vi "SetCommand.vi"(0 "reference in":refnum<class "Panel.lvclass">, 1 "Command.lvclass":refnum<class "Command.lvclass">, 5 "error in (no error)":errorcluster) -> (14 "reference out":refnum<class "Panel.lvclass">, 19 "error out":errorcluster)   [LabVIEW 2013]
uses:
  Panel.lvclass
  Command_class/Command.lvclass
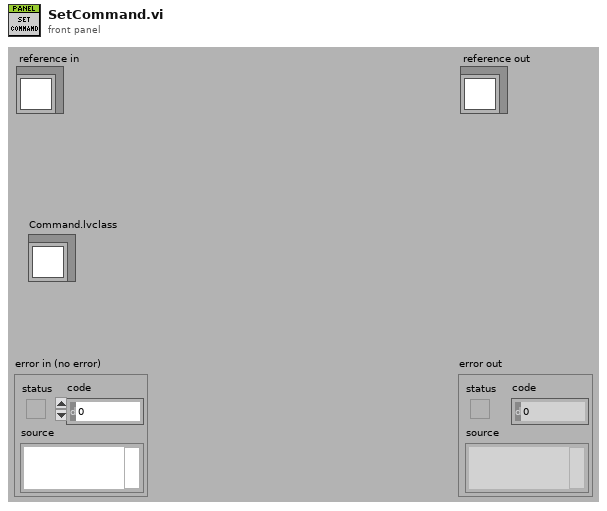
[diagram p1: front panel]
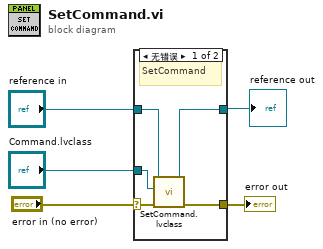
[diagram p0: block diagram]
diagram:
  n1 = case shown="无错误" "error in (no error)" {
    selector: "error in (no error)" -> [w7 w12]
    tunnel: [w6 w12] -> w4
    tunnel: [w9 w11] -> w2
    tunnel: "reference in" -> [w10 w11]
    tunnel: "Command.lvclass" -> [w8 _]
    frame No Error {
      # "SetCommand"
      n2 = call-dynamic "SetCommand.lvclass.vi"("error in (no error)"=w7, "Command.lvclass"=w8, "reference in"=w10) -> ("error out"=w6:errorcluster, "reference out"=w9:refnum<class "Panel.lvclass">)  [unwired: 7 in]
    }
    frame Error {
    }
  }
  "error out" <- w4
  "reference out" <- w2
